vi "conversion 2.vi"(10 "Channel Config":T1 {"Calibration matrix"."D.O."."K" format="%.6f"; "Calibration matrix"."D.O."."Temperature" format="%.2f"; "Calibration matrix"."pH scale"."Buffers"."V/T" format="%.5f"; "Calibration matrix"."pH scale"."Buffers"."Buffer" format="%.2f"; "Calibration matrix"."pH scale"."Temperature" format="%.2f"; "Calibration matrix"."offset (physical units)" format="%.5f"; "Calibration matrix"."correspondence table"."volts" format="%.4f"; "Calibration matrix"."correspondence table"."physical units" format="%.4f"; "Calibration matrix"."second channel" min=-1; "Calibration matrix"."offset (volts)" format="%.5f"; "Calibration matrix"."conversion matrix" format="%.4e"}, 11 "raw Data":T12 {"Sensor array" format="%.4f"; "Time" format="%<%I:%M:%S%2u %p\n%m/%d/%Y>T"}) -> (1 "Out of Range":bool[](array[boolean]), 2 "Calibrated data":T10 {"Sensor array"."scaled" format="%.2f"; "Sensor array"."voltage" format="%.4f"; "Time" format="%<%I:%M:%S%2u %p\n%m/%d/%Y>T"}, 3 "calibrated data":sgl[](array[numeric]) format="%.5f")   [LabVIEW 2019]
uses:
  Process Controller 3.0/Distributed Daq/raw data.ctl
  TCP DAQ/Sensor data.ctl
  DAQ configuration/sensor cluster.ctl
  Process Controller 3.0/Distributed Daq/Channel config.ctl
  DAQ configuration/channel identifier.ctl
  calib array.ctl
  conversion.ctl
  DAQ configuration/scale type.ctl
  correspondence table.ctl
  pH/pH scale.ctl
  Dissolved Oxygen/DO scale.ctl
  Spectrophotometer/Photometer calibration data.ctl
panel:
  # "C"
  # "kPa"
  # "C"
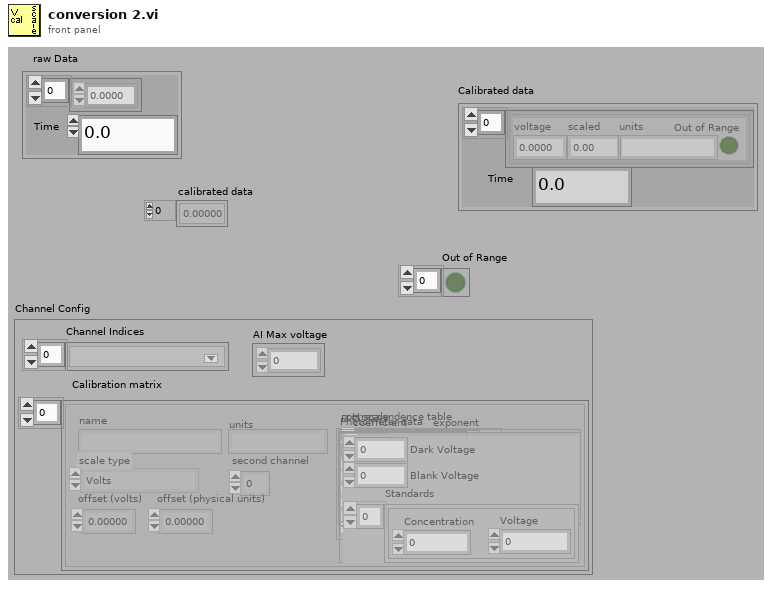
[diagram p1: front panel]
types:
  T1 = typedef "Channel config.ctl" = cluster{"Channel Indices":T2[], "AI Max voltage":dbl[], "Calibration matrix":T3}
  T2 = typedef "channel identifier.ctl" = u16
  T3 = typedef "calib array.ctl" = T4[]
  T4 = typedef "conversion.ctl" = cluster{"conversion matrix":sgl[][], "units":string, "name":string, "scale type":T5, "offset (volts)":dbl, "second channel":i8, "correspondence table":T6, "offset (physical units)":dbl, "pH scale":T7, "D.O.":T8, "Photometer data":T9}
  T5 = typedef "scale type.ctl" = enum16{"Volts", "Polynomial", "Correspondence Table", "pH", "Dissolved Oxygen", "Quadratic", "Photometer"}
  T6 = typedef "correspondence table.ctl" = cluster{"physical units":dbl, "volts":dbl}[]
  T7 = typedef "pH scale.ctl" = cluster{"Buffers":cluster{"Buffer":dbl, "Calibrated":bool, "V/T":dbl}[], "Temperature":dbl}
  T8 = typedef "DO scale.ctl" = cluster{"Temperature":dbl, "K":dbl, "barometric pressure":dbl}
  T9 = typedef "Photometer calibration data.ctl" = cluster{"Dark Voltage":dbl, "Blank Voltage":dbl, "Standards":cluster{"Concentration":dbl, "Voltage":dbl}[]}
  T10 = typedef "Sensor data.ctl" = cluster{" Sensor array":T11[], "Time":dbl}
  T11 = typedef "sensor cluster.ctl" = cluster{"voltage":sgl, "scaled":sgl, "units":string, "Out of Range":bool}
  T12 = typedef "raw data.ctl" = cluster{" Sensor array":sgl[], "Time":dbl}
  T13 = cluster{"voltage":sgl, dbl, "units":string, bool}[]
  T14 = cluster{cluster{"voltage":sgl, dbl, "units":string, bool}[], "Time":dbl}
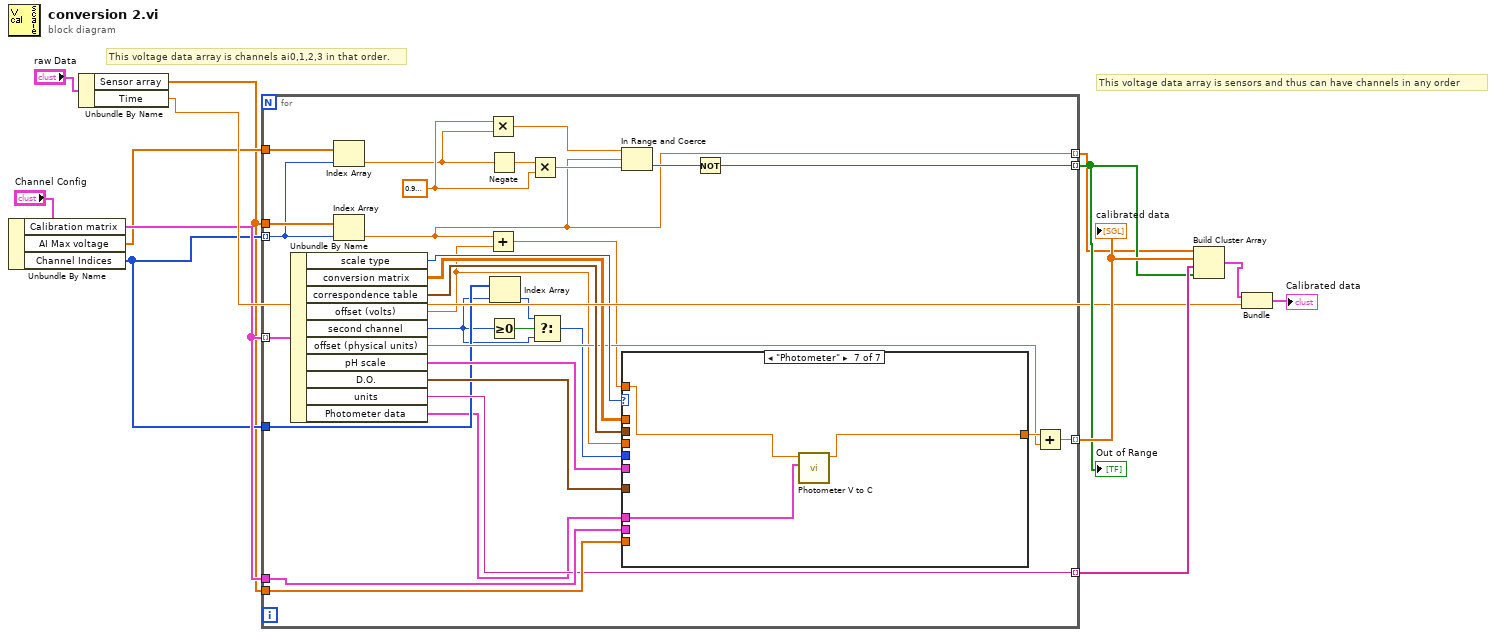
[diagram p0: block diagram]
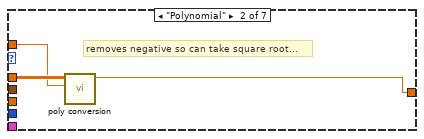
[diagram p3: hidden frame]
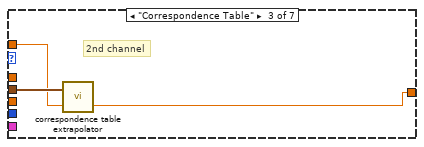
[diagram p4: hidden frame]
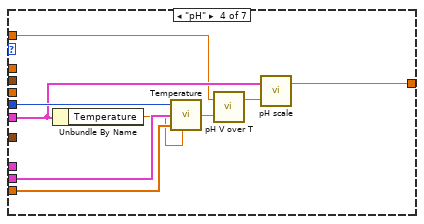
[diagram p5: hidden frame]
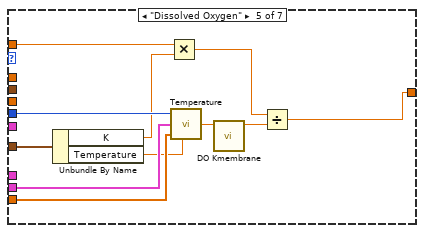
[diagram p6: hidden frame]
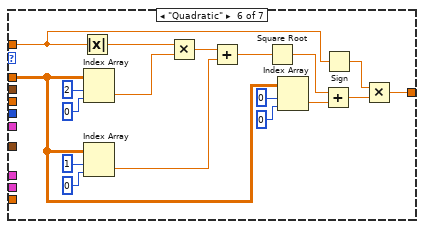
[diagram p7: hidden frame]
diagram:
  # "This voltage data array is sensors and thus can have channels in any order"
  # "This voltage data array is channels ai0,1,2,3 in that order."
  n1 = Unbundle By Name("Channel Config") -> ("Calibration matrix"=w5:T3, "AI Max voltage"=w3:dbl[], "Channel Indices"=w4:T2[])
  n2 = Unbundle By Name("raw Data") -> ("Sensor array"=w2:sgl[], "Time"=w8:dbl)
  n3 = for {
    tunnel: w5 -> [w29] mode=indexing
    tunnel: w2 -> [w23]
    tunnel: w2 -> [w39]
    tunnel: [w38] -> w13 mode=indexing
    tunnel: [w33] -> w11 mode=indexing
    tunnel: w4 -> [w22] mode=indexing
    tunnel: w5 -> [w30]
    tunnel: [w24] -> w12 mode=indexing
    tunnel: w4 -> [w21]
    tunnel: w3 -> [w20]
    tunnel: [w19] -> w1 mode=indexing
    w37 = sgl 0.99 ("x")
    n4 = Unbundle By Name(w29) -> ("scale type"=w43:T5, "conversion matrix"=w44:sgl[][], "correspondence table"=w42:T6, "offset (volts)"=w28:dbl, "second channel"=w17:i8, "offset (physical units)"=w40:dbl, "pH scale"=w32:T7, "D.O."=w31:T8, "units"=w24:string, "Photometer data"=w14:T9)
    n5 = Index Array(array=w20, index=w22) -> (element=w26:dbl)
    n6 = Index Array(array=w23, index=w22) -> (element=w19:sgl)
    n7 = Multiply(x=w37, y=w26) -> (x*y=w36:dbl)
    n8 = Add(x=w19, y=w28) -> (x+y=w27:dbl)
    n9 = Negate(x=w26) -> (-x=w25:dbl)
    n10 = Greater Or Equal To 0?(x=w17) -> (x >= 0?=w18:bool)
    n11 = Index Array(array=w21, index=w17) -> (element=w16:T2)
    n12 = Multiply(x=w25, y=w37) -> (x*y=w35:dbl)
    n13 = Select(t=w16, s=w18, f=w17) -> (s? t:f=w15:T2)
    n14 = In Range and Coerce(upper limit=w36, x=w19, lower limit=w35) -> (In Range?=w34:bool)  [unwired: 1 out]
    n15 = case shown="\"Photometer\"" w43 {
      tunnel: w44 -> [_ w48 _ _ _ w75 _]
      tunnel: [w45 w47 w50 w54 w71 w73 w91] -> w41
      tunnel: w42 -> [_ _ w51 _ _ _ _]
      tunnel: w28 -> [_ _ _ _ _ _ _]
      tunnel: w15 -> [_ _ _ w60 w67 _ _]
      tunnel: w30 -> [_ _ _ w59 w69 _ _]
      tunnel: w39 -> [_ _ _ w58 w68 _ _]
      tunnel: w32 -> [_ _ _ w55 _ _ _]
      tunnel: w31 -> [_ _ _ _ w65 _ _]
      tunnel: w27 -> [w45 w46 w49 w52 w61 w72 w92]
      tunnel: w14 -> [_ _ _ _ _ _ w90]
      frame "Volts", Default {
      }
      frame "Polynomial" {
        # "removes negative so can take square root..."
        n16 = call "poly conversion.vi"("Volts"=w46, "conversion matrix"=w48) -> ("Calibrated value"=w47:dbl)  [unwired: 9 in]
      }
      frame "Correspondence Table" {
        # "2nd channel"
        n17 = call "correspondence table extrapolator.vi"("Volts"=w49, "correspondence table"=w51) -> ("scaled"=w50:dbl)  [unwired: 1 out]
      }
      frame "pH" {
        n18 = Unbundle By Name(w55) -> ("Temperature"=w56:dbl)
        n19 = call "Temperature.vi"("second channel"=w60, "selected calibration array"=w59, "voltage data"=w58, "Default Temperature (C)"=w56) -> ("Temperature (C)"=w57:dbl)  [unwired: 1 in]
        n20 = call "pH V over T.vi"("Temperature"=w57, "Voltage"=w52) -> ("V/T"=w53:dbl)  [unwired: 1 out]
        n21 = call "pH scale.vi"("V/T"=w53, "pH scale"=w55) -> ("pH"=w54:dbl)  [unwired: 1 out]
      }
      frame "Dissolved Oxygen" {
        n22 = Unbundle By Name(w65) -> ("K"=w63:dbl, "Temperature"=w64:dbl)
        n23 = Multiply(x=w61, y=w63) -> (x*y=w62:dbl)
        n24 = call "Temperature.vi"("second channel"=w67, "selected calibration array"=w69, "voltage data"=w68, "Default Temperature (C)"=w64) -> ("Temperature (C)"=w66:dbl)  [unwired: 1 in]
        n25 = call "DO Kmembrane.vi"("Temperature (C)"=w66) -> ("Kmembrane"=w70:dbl)  [unwired: 10 in]
        n26 = Divide(x=w62, y=w70) -> (x/y=w71:dbl)
      }
      frame "Quadratic" {
        n27 = Absolute Value(x=w72) -> (abs(x)=w85:dbl)
        n28 = Index Array(array=w75, index (row)=2 ("Index"), index (col)=0 ("Disabled Index (col)")) -> (element=w81:sgl)
        n29 = Index Array(array=w75, index (row)=1 ("Index"), index (col)=0 ("Disabled Index (col)")) -> (element=w78:sgl)
        n30 = Multiply(x=w85, y=w81) -> (x*y=w87:dbl)
        n31 = Add(x=w87, y=w78) -> (x+y=w86:dbl)
        n32 = Square Root(x=w86) -> (sqrt(x)=w84:dbl)
        n33 = Index Array(array=w75, index (row)=0 ("Index"), index (col)=0 ("Disabled Index (col)")) -> (element=w74:sgl)
        n34 = Add(x=w84, y=w74) -> (x+y=w83:dbl)
        n35 = Sign(1:w72) -> (0:w82:dbl)
        n36 = Multiply(x=w82, y=w83) -> (x*y=w73:dbl)
      }
      frame "Photometer" {
        n37 = call "Photometer V to C.vi"("Photometer data in"=w90, "Volts"=w92) -> ("Concentration"=w91:dbl)  [unwired: 8 in, 1 out]
      }
    }
    n38 = Not(x=w34) -> (.not. x?=w33:bool)
    n39 = Add(x=w41, y=w40) -> (x+y=w38:dbl)
  }
  "calibrated data" <- w13
  "Out of Range" <- w11
  n40 = Build Cluster Array(w1, w13, w12, w11) -> (w9:T13)
  n41 = Bundle(w9, "Time"=w8) -> (→"Calibrated data":T14)  [unwired: 1 in]
